vi "3DObject.vi"() -> ()   [LabVIEW 2011]
uses:
  <vilib>/picture/3D Picture Control/NI_3D Picture Control.lvlib
panel:
  in  "stop":bool
  out "3D Picture":refnum<vi>(3d-picture)
  in  "Zrad":dbl(slide) scale=0.0..10.0
  out "Slide 4":dbl
  in  "Yrad":dbl(slide) scale=0.0..10.0
  out "Slide 3":dbl
  out "Slide 2":dbl
  in  "Xrad":dbl(slide) scale=0.0..10.0
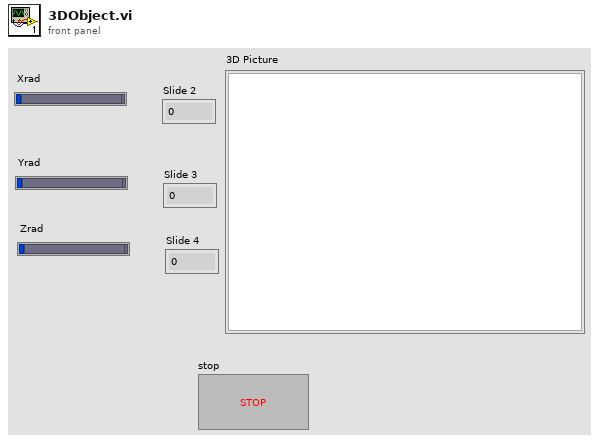
[diagram p1: front panel]
types:
  T1 = cluster{"Red":sgl, "Green":sgl, "Blue":sgl, "Alpha":sgl}
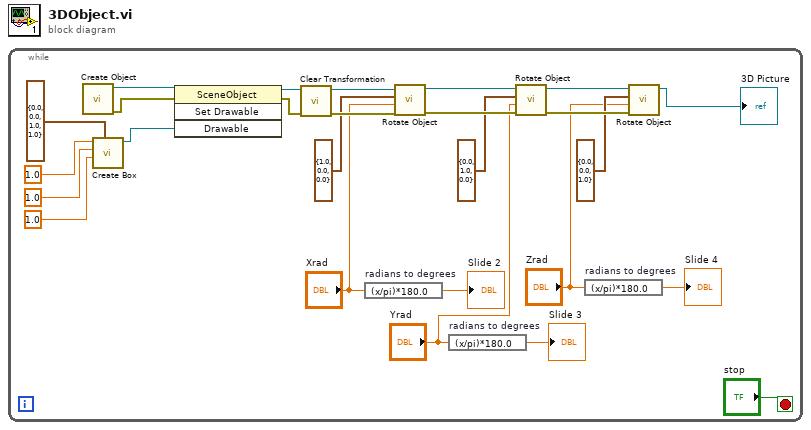
[diagram p0: block diagram]
diagram:
  n1 = while {
    stop <- "stop" stop-if-true
    n2 = call <vilib>:"Create Object.vi"() -> ("error out"=w21:errorcluster, "Scene:New Object"=w22:refnum<vi>)  [unwired: 10 in]
    n3 = call <vilib>:"Create Box.vi"("Color"=T1 {"Red"=0.0, "Green"=0.0, "Blue"=1.0, "Alpha"=1.0}, "Length Z"=sgl 1.0, "Length Y"=sgl 1.0, "Length X"=sgl 1.0) -> ("New Box Refnum"=w20:refnum<vi>)  [unwired: 6 in, 1 out]
    n4 = invoke class="SceneObject" method="Set Drawable"(reference=w22, error in=w21, "Drawable"=w20) -> (reference out=w19:refnum<vi>, error out=w18:errorcluster)  [unwired: 1 in, 2 out]
    n5 = call <vilib>:"Clear Transformation.vi"("error in (no error)"=w18, "Object Refnum In"=w19) -> ("error out"=w17:errorcluster, "Object Refnum Out"=w16:refnum<vi>)  [unwired: 8 in]
    n6 = expression code="(x/pi)*180.0" "radians to degrees"("Xrad") -> (→"Slide 2":dbl)
    n7 = call <vilib>:"Rotate Object.vi"("error in (no error)"=w17, "Angle"="Xrad", "Axis"=cluster{"X":sgl, "Y":sgl, "Z":sgl} {"X"=1.0, "Y"=0.0, "Z"=0.0}, "Scene.Object In"=w16) -> ("error out"=w15:errorcluster, "Scene.Object Out"=w14:refnum<vi>)  [unwired: 6 in]
    n8 = expression code="(x/pi)*180.0" "radians to degrees"("Yrad") -> (→"Slide 3":dbl)
    n9 = call <vilib>:"Rotate Object.vi"("error in (no error)"=w15, "Angle"="Yrad", "Axis"=cluster{"X":sgl, "Y":sgl, "Z":sgl} {"X"=0.0, "Y"=1.0, "Z"=0.0}, "Scene.Object In"=w14) -> ("error out"=w13:errorcluster, "Scene.Object Out"=w12:refnum<vi>)  [unwired: 6 in]
    n10 = expression code="(x/pi)*180.0" "radians to degrees"("Zrad") -> (→"Slide 4":dbl)
    n11 = call <vilib>:"Rotate Object.vi"("error in (no error)"=w13, "Angle"="Zrad", "Axis"=cluster{"X":sgl, "Y":sgl, "Z":sgl} {"X"=0.0, "Y"=0.0, "Z"=1.0}, "Scene.Object In"=w12) -> ("Scene.Object Out"=→"3D Picture":refnum<vi>)  [unwired: 6 in, 1 out]
  }
